vi "Setup UI.vi"(8 "error in (no error)":errorcluster, 10 "Set UI to input? (F)":bool, 11 "Reader in":refnum<class "Reader.lvclass">) -> (0 "error out":errorcluster, 3 "Reader out":refnum<class "Reader.lvclass">)   [LabVIEW 2012, in "Reader.lvclass"]
doc: "Setup UI constructs an object -- populates its member fields -- from a front panel the user can see. The VI should be as simple as possible so that a UI loop can poll it continuously for updates. \n\nThe VI is designed to be used as a subPanel within another VI. Wire true to \"Set UI to input\" only on the first call, just after inserting this VI into a subPanel, to populate its controls with the class's current values.\n\nSetup UI is distinct from the class constructor. Class constructors are not polymorphic, yet configure dialogs need to configure objects without knowing their type -- and polymorphism is the necessary solution. Thus, Setup UI is a polymorphic class constructor. This continously polled \"Setup UI\" concept is a kludge: a better idea would be an XControl, but those require a steeper learning curve."
uses:
  Reader.lvclass
  Reader.lvclass/Reader.ctl
  Instruments/Utility Classes/Readable/Readable.lvclass
panel:
  in  "Dwell Time":dbl[unit]
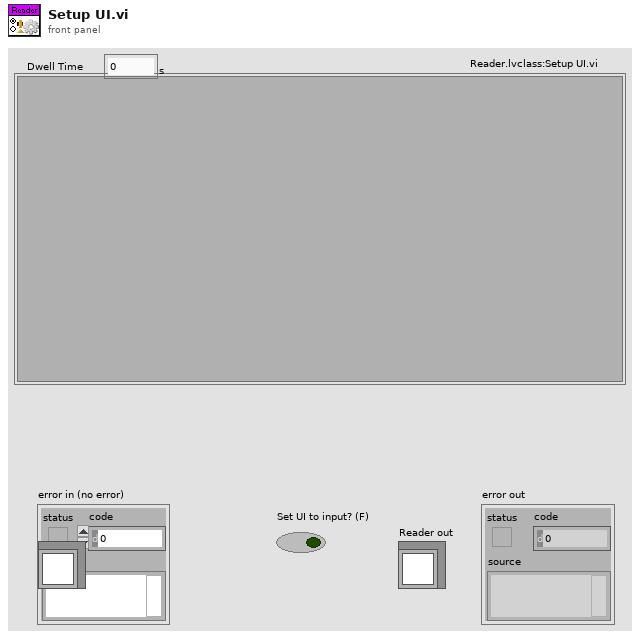
[diagram p1: front panel]
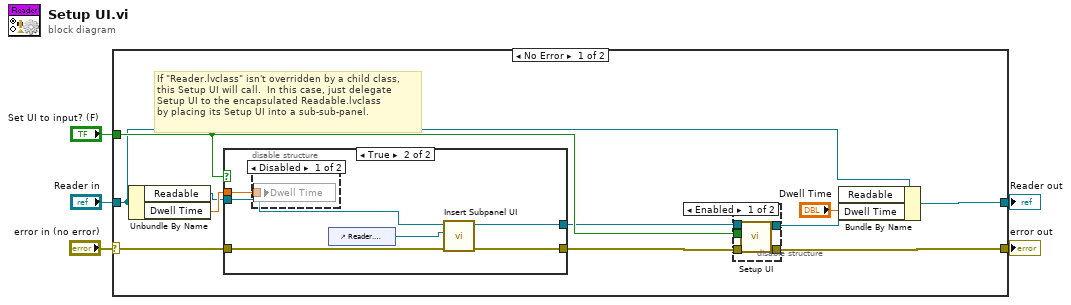
[diagram p0: block diagram]
diagram:
  n1 = case shown="No Error" "error in (no error)" {
    selector: "error in (no error)" -> [w15 w34]
    tunnel: [w13 w34] -> w4
    tunnel: [w16 w33] -> w1
    tunnel: "Reader in" -> [w9 w33]
    tunnel: "Set UI to input? (F)" -> [w14 _]
    frame No Error {
      # "If \"Reader.lvclass\" isn't overridden by a child class,\nthis Setup UI will call.  In this case, just delegate\nSetup UI to the encapsulated Readable.lvclass\nby placing its Setup UI into a sub-sub-panel."
      n2 = Unbundle By Name(w9) -> ("Readable"=w8:refnum<class "Readable.lvclass">, "Dwell Time"=w10:dbl[unit])
      n3 = case shown="True" w14 {
        tunnel: [w24 w30] -> w7
        tunnel: w15 -> [w25 w29]
        tunnel: [w25 w28] -> w12
        tunnel: w10 -> [_ w27]
        tunnel: w8 -> [w24 w26]
        frame False {
        }
        frame True {
          n4 = disable-structure shown="Disabled" {
            disable-tunnel: w27 -> [w32 _]
            frame Disabled {
              n5 = local write "Dwell Time"(w32) -> ()
            }
            frame Enabled {
            }
          }
          n6 = control-ref of="Reader.lvclass:Setup UI.vi"() -> (w31:refnum<vi>)
          n7 = call "Insert Subpanel UI.vi"("error in (no error)"=w29, "Subpanel in"=w31, "LabVIEW Object"=w26) -> ("error out"=w28:errorcluster, "LabVIEW Object out"=w30:refnum<class "Readable.lvclass">)  [unwired: 7 out]
        }
      }
      n8 = disable-structure shown="Enabled" {
        disable-tunnel: w14 -> [w21 _]
        disable-tunnel: [w20 w22] -> w13
        disable-tunnel: w12 -> [w19 w22]
        disable-tunnel: w7 -> [w18 w23]
        disable-tunnel: [w17 w23] -> w6
        frame Enabled {
          n9 = call-dynamic "Setup UI.vi"("error in (no error)"=w19, "Set UI to input? (F)"=w21, "Instrument in"=w18) -> ("error out"=w20:errorcluster, "Instrument out"=w17:refnum<class "Readable.lvclass">)  [unwired: 7 out]
        }
        frame Disabled {
        }
      }
      n10 = Bundle By Name(cluster=w9, "Readable"=w6, "Dwell Time"="Dwell Time") -> (w16:refnum<class "Reader.lvclass">)
    }
    frame Error {
    }
  }
  "error out" <- w4
  "Reader out" <- w1
